vi "Create Mesh form Verticies.vi"(8 "error in (no error)":errorcluster, 10 "Verticies":T1[](array[typedef]), 11 "Object Name":string) -> (0 "error out":errorcluster, 3 "SceneObject out":refnum<vi>)   [LabVIEW 2020, in "g_ar_toolkit.ar.lvlib"]
uses:
  g_ar_toolkit.ar.lvlib
  Vertex Descriptor.ctl
  <vilib>/Utility/miscctls.llb/LV3DPointTypeDef.ctl
  <vilib>/Utility/miscctls.llb/LVRGBAColorTypeDef.ctl
  <vilib>/picture/3D Picture Control/Object/Create Object (drawable).vi
  <vilib>/picture/3D Picture Control/NI_3D Picture Control.lvlib
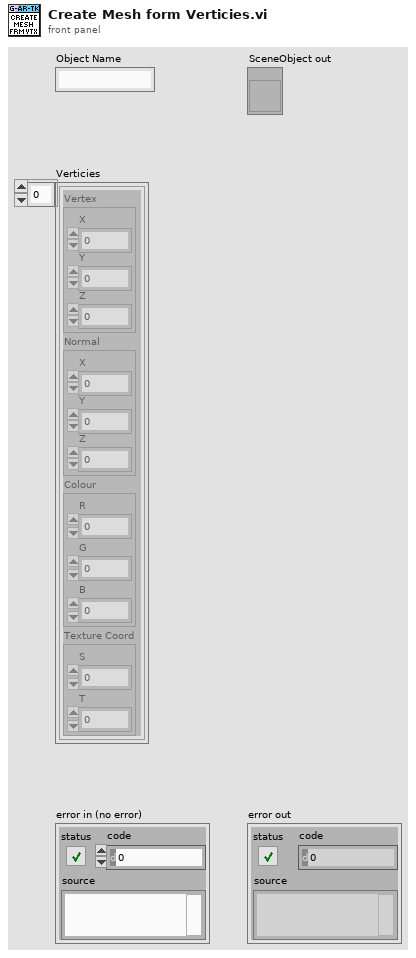
[diagram p1: front panel]
types:
  T1 = typedef "g_ar_toolkit.ar.lvlib/Vertex Descriptor.ctl" = cluster{"Vertex":T2, "Normal":T2, "Colour":cluster{"R":sgl, "G":sgl, "B":sgl}, "Texture Coord":cluster{"S":sgl, "T":sgl}}
  T2 = typedef "LV3DPointTypeDef.ctl" = cluster{"X":sgl, "Y":sgl, "Z":sgl}
  T3 = enum16{"Overall", "Per Primitive", "Per Vertex", "Binding Off"}
  T4 = enum16{"Points", "Lines", "Line Strip", "Line Loop", "Triangles", "Triangle Strip", "Triangle Fan", "Quads", "Quad Strip", "Polygon"}
  T5 = typedef "LVRGBAColorTypeDef.ctl" = cluster{"Red":sgl, "Green":sgl, "Blue":sgl, "Alpha":sgl}
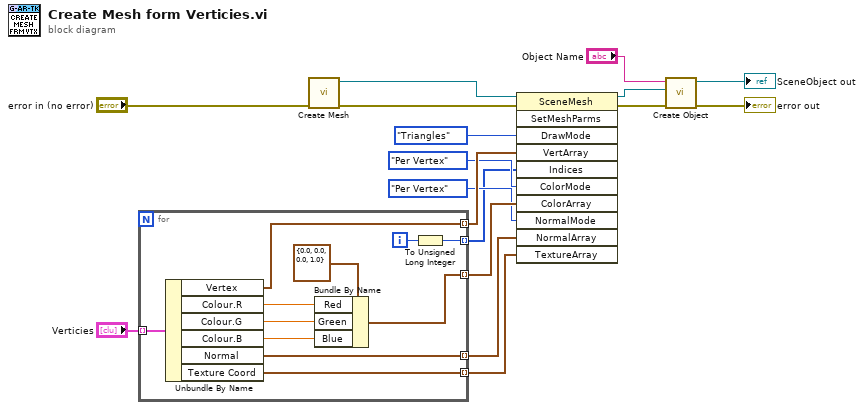
[diagram p0: block diagram]
diagram:
  n1 = for {
    tunnel: "Verticies" -> [w28] mode=indexing
    tunnel: [w27] -> w17 mode=indexing
    tunnel: [w25] -> w4 mode=indexing
    tunnel: [w24] -> w14 mode=indexing
    tunnel: [w23] -> w12 mode=indexing
    tunnel: [w22] -> w11 mode=indexing
    i -> [w26]
    n2 = Unbundle By Name(w28) -> ("Vertex"=w27:T2, "Colour.R"=w21:sgl, "Colour.G"=w20:sgl, "Colour.B"=w19:sgl, "Normal"=w23:T2, "Texture Coord"=w22:cluster{"S":sgl, "T":sgl})
    n3 = Bundle By Name(cluster=T5 {"Red"=0.0, "Green"=0.0, "Blue"=0.0, "Alpha"=1.0} ("Color"), "Red"=w21, "Green"=w20, "Blue"=w19) -> (w24:T5)
    n4 = To Unsigned Long Integer(number=w26) -> (unsigned 32bit integer=w25:u32)
  }
  n5 = call <vilib>:"Create Mesh.vi"("error in (no error)"="error in (no error)") -> ("error out"=w6:errorcluster, "New Mesh Refnum"=w3:refnum<vi>)  [unwired: 9 in]
  n6 = invoke class="SceneMesh" method="SetMeshParms"(reference=w3, error in=w6, "DrawMode"=T4."Triangles" ("Draw Mode"), "VertArray"=w17, "Indices"=w4, "ColorMode"=T3."Per Vertex" ("Color Binding Mode"), "ColorArray"=w14, "NormalMode"=T3."Per Vertex" ("Normal Binding Mode"), "NormalArray"=w12, "TextureArray"=w11) -> (reference out=w10:refnum<vi>, error out=w5:errorcluster)  [unwired: 1 in, 9 out]
  n7 = call-poly <vilib>:"Create Object.vi"("error in (no error)"=w5, "Geometry"=w10, "Name"="Object Name") -> ("error out"=→"error out":errorcluster, "Scene:New Object"=→"SceneObject out":refnum<vi>)  [unwired: 7 in]
